vi "msg_calibragem.vi"(8 "error in (no error)":errorcluster, 9 "Enable":bool=TRUE, 10 "Message":string="Iniciaremos agora o processo de calibragem comandado pelo Bob.") -> (0 "error out":errorcluster, 2 "Ok!":bool)   [LabVIEW 2013]
doc: "Displays a standard dialog box that contains an alert or a message for users.\n--------------------\n\nThis Express VI is configured as follows:\n\nMessage: Iniciaremos agora o processo de calibragem comandado pelo Bob."
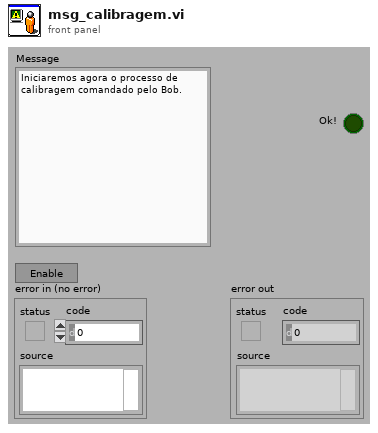
[diagram p1: front panel]
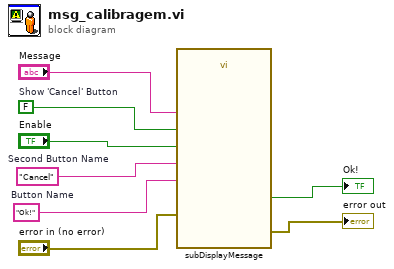
[diagram p0: block diagram]
diagram:
  w3 = "Ok!"  # Button Name
  w4 = "Cancel"  # Second Button Name
  w6 = FALSE  # Show 'Cancel' Button
  n1 = call <vilib>:"subDisplayMessage.vi"("Second Button Name"=w4, "Button Name"=w3, "error in (no error)"="error in (no error)", "Enable Message"="Enable", "Show 'Cancel' Button"=w6, "Message to Display"="Message") -> ("error out"=→"error out":errorcluster, "OK?"=→"Ok!":bool)  [unwired: 4 in]
